vi "Get LakeShore 340 Set Point.vi"(8 "error in (no error)":errorcluster, 10 "Output #":i32=1, 11 "VISA Resource Name":refnum<visa-resource-name>) -> (0 "error out":errorcluster, 2 "Set point":dbl, 3 "VISA Resource Name Out":refnum<visa-resource-name>)   [LabVIEW 2021]
uses:
  GPIB/VISA  Send Receive.vi
  Simple VISA Reader/Simple VISA Reader Driver.lvclass
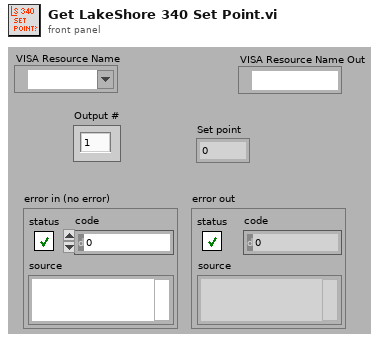
[diagram p1: front panel]
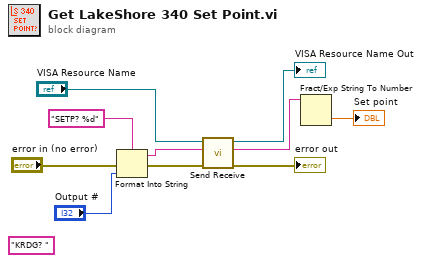
[diagram p0: block diagram]
diagram:
  (unwired) "KRDG? " ("data string in")
  n1 = Format Into String(format string="SETP? %d" ("data string"), error in="error in (no error)", "Output #") -> (resulting string=w1:string, error out=w4:errorcluster)  [unwired: 1 in]
  n2 = call-poly "Send Receive.vi"("error in (no error)"=w4, "data string in"=w1, "VISA Resource Name"="VISA Resource Name") -> ("error out"=→"error out":errorcluster, "data string out"=w9:string, "VISA Resource Name Out"=→"VISA Resource Name Out":refnum<visa-resource-name>)  [unwired: 6 in]
  n3 = Fract/Exp String To Number(string=w9) -> (number=→"Set point":dbl)  [unwired: 4 out]
